vi "知乎日报.vi"() -> ()   [LabVIEW 2012]
panel:
  in  "关于作者":bool
  in  "刷新":bool
  out "stories":T1(array[cluster])
  out "top_stories":cluster{"字符串 2":string, "二维图片":picture}[](array[cluster])
  out "title with pic":cluster{"字符串 2":string, "二维图片":picture}[](array[cluster])
  in  "WebBrowser":refnum<k7>(container) caption="网页浏览器"
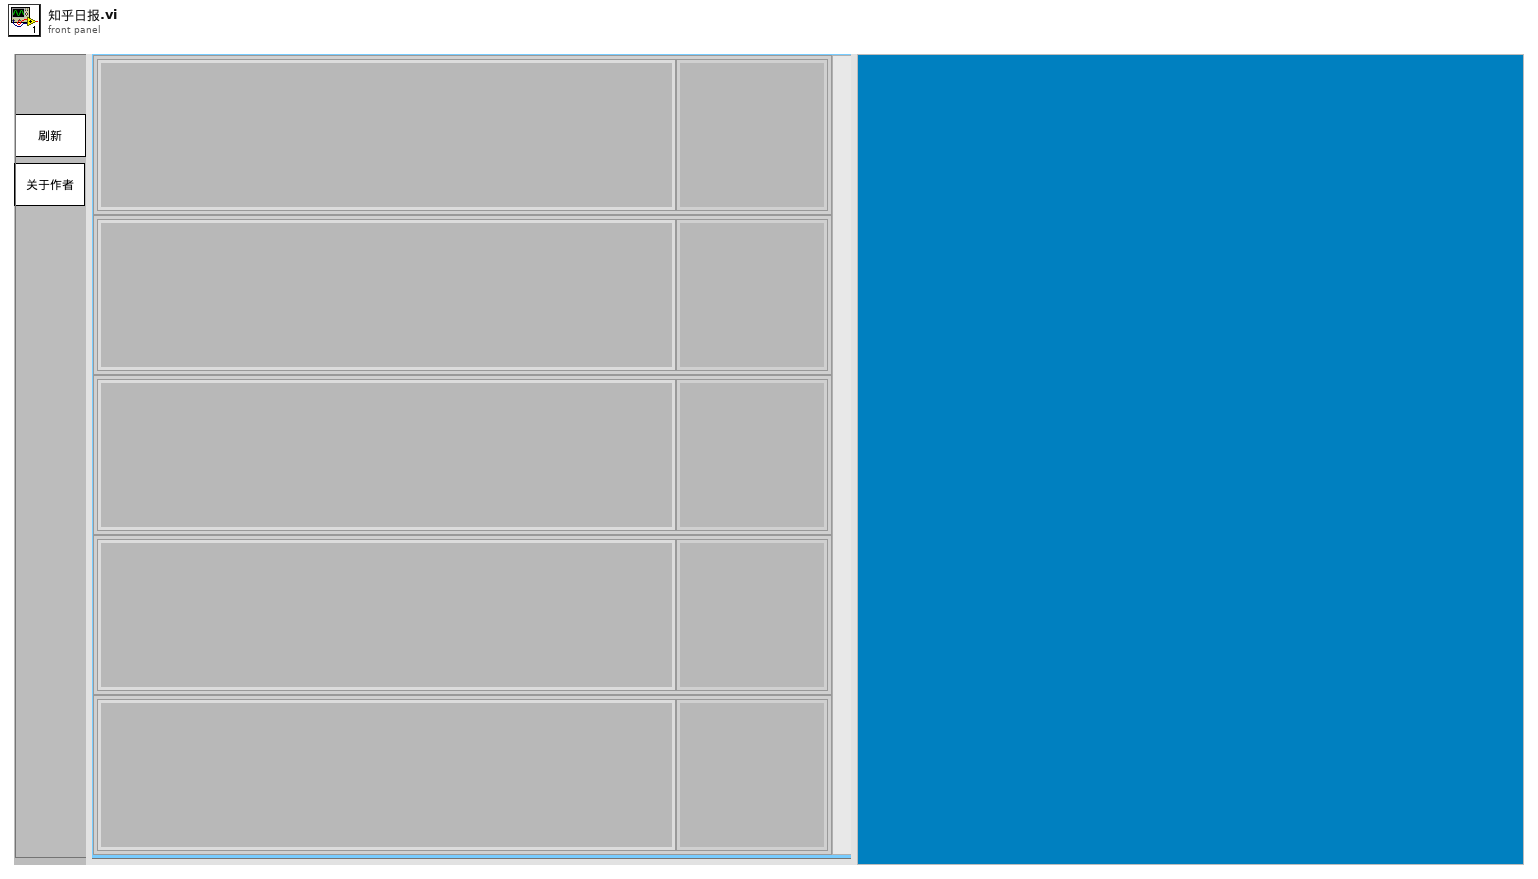
[diagram p1: front panel]
types:
  T1 = cluster{"images":string, "type":i32, "id":i64, "ga_prefix":string, "title":string}[]
  T2 = cluster{"images":string, "type":i32, "id":i64, "ga_prefix":string, "title":string}
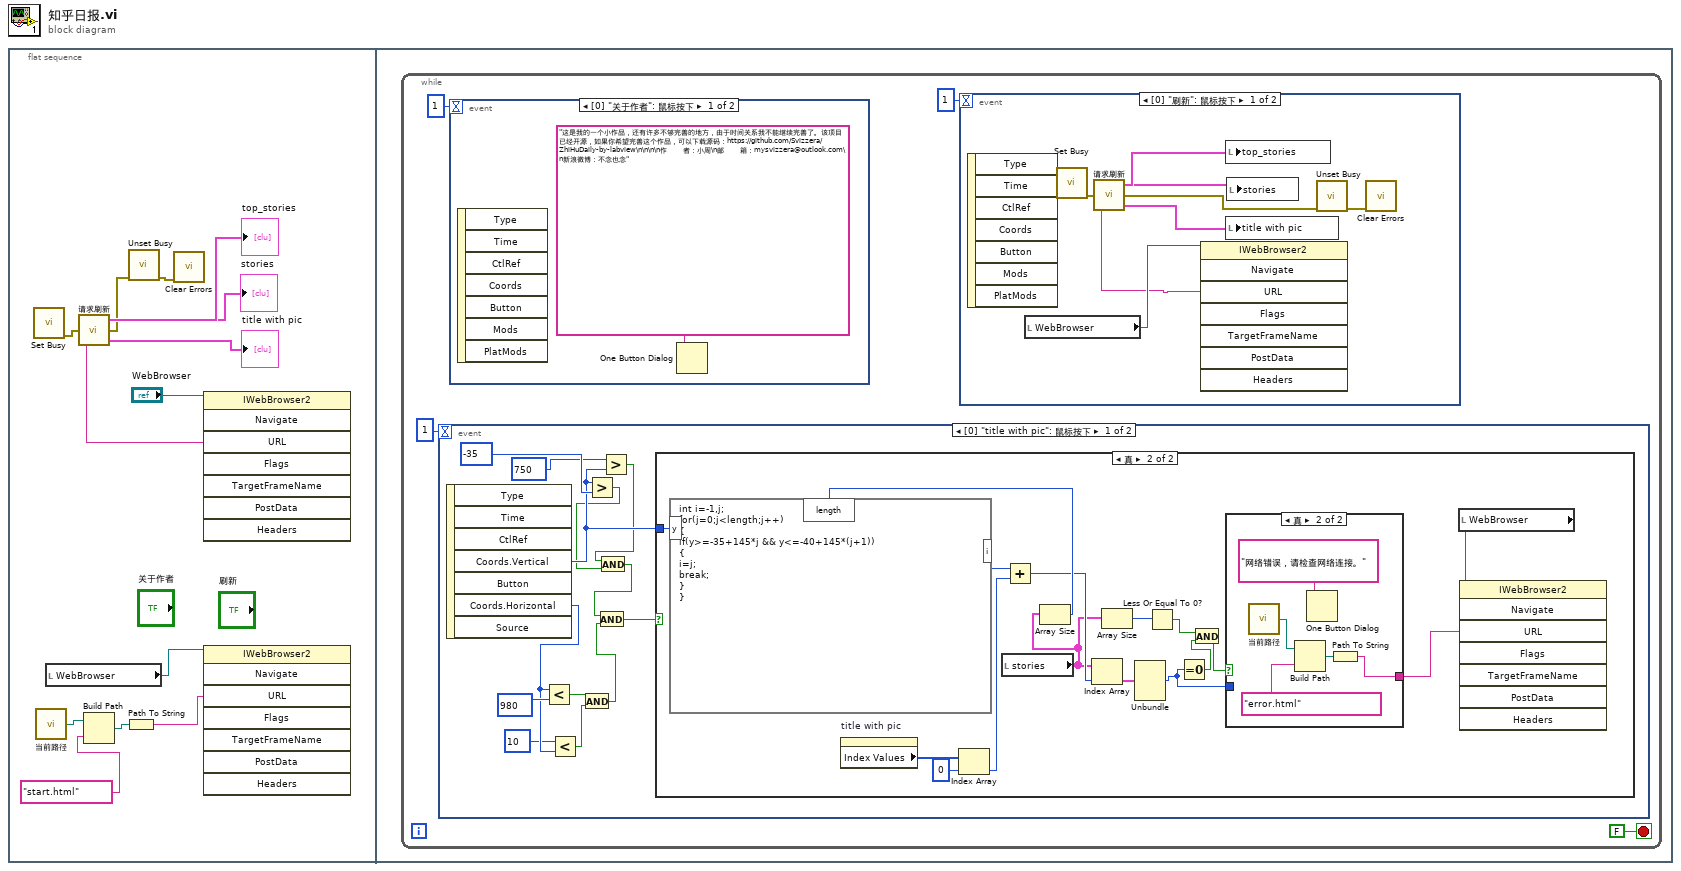
[diagram p0: block diagram]
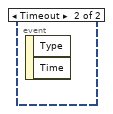
[diagram p2: hidden frame]
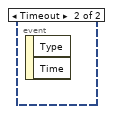
[diagram p3: hidden frame]
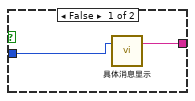
[diagram p5: hidden frame]
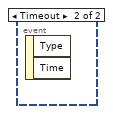
[diagram p6: hidden frame]
diagram:
  n1 = flat-sequence {
    frame #0 {
      n2 = call <vilib>:"Set Busy.vi"() -> ("error out"=w9:errorcluster)  [unwired: 10 in, 1 out]
      n3 = call "当前路径.vi"() -> ("路径"=w4:path)
      n4 = local read "WebBrowser"() -> (w5:refnum<k7>)
      n5 = call "请求刷新.vi"("Error Out"=w9) -> ("title with pic"=→"title with pic":cluster{"字符串 2":string, "二维图片":picture}[], "error out"=w7:errorcluster, "stories"=→"stories":T1, "URL"=w6:string, "top_stories"=→"top_stories":cluster{"字符串 2":string, "二维图片":picture}[])
      n6 = Build Path(base path=w4, name or relative path="start.html") -> (appended path=w2:path)
      n7 = Path To String(path=w2) -> (string=w1:string)
      n8 = call <vilib>:"Unset Busy.vi"("error in (no error)"=w7) -> ("error out"=w8:errorcluster)  [unwired: 10 in]
      n9 = call <vilib>:"Clear Errors.vi"("error in (no error)"=w8) -> ()  [unwired: 6 in, 1 out]
      n10 = invoke class="IWebBrowser2" method="Navigate"(reference="WebBrowser", "URL"=w6) -> ()  [unwired: 6 in, 8 out]
      n11 = invoke class="IWebBrowser2" method="Navigate"(reference=w5, "URL"=w1) -> ()  [unwired: 6 in, 8 out]
    }
    frame #1 {
      n12 = while {
        stop <- FALSE stop-if-true
        n13 = event shown="[0] \"title with pic\": 鼠标按下" {
          selector: _ -> [_ _]
          dyn-events: _ -> [_ _]
          timeout: 1 -> [_ _]
          event "title with pic": Mouse Down {
            n14 = event-data() -> ("Coords.Vertical"=w36:i32, "Coords.Horizontal"=w31:i32)  [unwired: 1 in, 5 out]
            n15 = Less?(x=w31, y=980) -> (x < y?=w29:bool)
            n16 = Less?(x=10, y=w31) -> (x < y?=w28:bool)
            n17 = And(x=w29, y=w28) -> (x .and. y?=w27:bool)
            n18 = Greater?(x=w36, y=-35) -> (0:w33:bool)
            n19 = Greater?(x=750, y=w36) -> (0:w34:bool)
            n20 = And(x=w34, y=w33) -> (x .and. y?=w32:bool)
            n21 = And(x=w32, y=w27) -> (x .and. y?=w37:bool)
            n22 = case shown="真" w37 {
              tunnel: w36 -> [_ w48]
              frame False {
              }
              frame True {
                n23 = property on="title with pic" class="Arr (严格)"() -> ("Index Values"=w51:u32[])  [unwired: 2 in, 2 out]
                n24 = Index Array(array=w51, index=0) -> (element=w49:u32)
                n25 = local read "stories"() -> (w45:T1)
                n26 = Array Size(array=w45) -> (size(s)=w53:i32)
                n27 = formula code="int i=-1,j;\nfor(j=0;j<length;j++)\n{\nif(y>=-35+145*j && y<=-40+145*(j+1))\n{\ni=j;\nbreak;\n}\n}"("y"=w48, "length"=w53) -> ("i"=w52:i32)
                n28 = Add(x=w52, y=w49) -> (x+y=w47:u32)
                n29 = Index Array(array=w45, index=w47) -> (element=w46:T2)
                n30 = Array Size(array=w45) -> (size(s)=w44:i32)
                n31 = Unbundle(w46) -> ("id"=w54:i64)  [unwired: 4 out]
                n32 = Less Or Equal To 0?(x=w44) -> (x <= 0?=w42:bool)
                n33 = Equal To 0?(x=w54) -> (x = 0?=w41:bool)
                n34 = And(x=w42, y=w41) -> (x .and. y?=w43:bool)
                n35 = case shown="真" w43 {
                  tunnel: w54 -> [w57 _]
                  tunnel: [w56 w58] -> w40
                  frame False {
                    n36 = call "具体消息显示.vi"("ID"=w57) -> ("html_url"=w56:string)  [unwired: 2 in]
                  }
                  frame True {
                    n37 = call "当前路径.vi"() -> ("路径"=w60:path)
                    n38 = Build Path(base path=w60, name or relative path="error.html") -> (appended path=w62:path)
                    n39 = One Button Dialog(message="网络错误，请检查网络连接。") -> ()  [unwired: 1 in, 1 out]
                    n40 = Path To String(path=w62) -> (string=w58:string)
                  }
                }
                n41 = local read "WebBrowser"() -> (w55:refnum<k7>)
                n42 = invoke class="IWebBrowser2" method="Navigate"(reference=w55, "URL"=w40) -> ()  [unwired: 6 in, 8 out]
              }
            }
          }
          event Timeout {
            n43 = event-data() -> ()  [unwired: 1 in, 2 out]
          }
        }
        n44 = event shown="[0] \"关于作者\": 鼠标按下" {
          selector: _ -> [_ _]
          dyn-events: _ -> [_ _]
          timeout: 1 -> [_ _]
          event "关于作者": Mouse Down {
            n45 = event-data() -> ()  [unwired: 1 in, 7 out]
            n46 = One Button Dialog(message="这是我的一个小作品，还有许多不够完善的地方，由于时间关系我不能继续完善了。该项目已经开源，如果你希望完善这个作品，可以下载源码：https://github.com/Svizzera/ZhiHuDaily-by-labview\n\n\n\n作        者：小周\n邮        箱：mysvizzera@outlook.com\n新浪微博：不念也念") -> ()  [unwired: 1 in, 1 out]
          }
          event Timeout {
            n47 = event-data() -> ()  [unwired: 1 in, 2 out]
          }
        }
        n48 = event shown="[0] \"刷新\": 鼠标按下" {
          selector: _ -> [_ _]
          dyn-events: _ -> [_ _]
          timeout: 1 -> [_ _]
          event "刷新": Mouse Down {
            n49 = event-data() -> ()  [unwired: 1 in, 7 out]
            n50 = local read "WebBrowser"() -> (w25:refnum<k7>)
            n51 = call <vilib>:"Set Busy.vi"() -> ("error out"=w20:errorcluster)  [unwired: 10 in, 1 out]
            n52 = call "请求刷新.vi"("Error Out"=w20) -> ("title with pic"=w22:cluster{"字符串 2":string, "二维图片":picture}[], "error out"=w19:errorcluster, "stories"=w23:T1, "URL"=w18:string, "top_stories"=w24:cluster{"字符串 2":string, "二维图片":picture}[])
            n53 = invoke class="IWebBrowser2" method="Navigate"(reference=w25, "URL"=w18) -> ()  [unwired: 6 in, 8 out]
            n54 = local write "top_stories"(w24) -> ()
            n55 = local write "title with pic"(w22) -> ()
            n56 = local write "stories"(w23) -> ()
            n57 = call <vilib>:"Unset Busy.vi"("error in (no error)"=w19) -> ("error out"=w21:errorcluster)  [unwired: 10 in]
            n58 = call <vilib>:"Clear Errors.vi"("error in (no error)"=w21) -> ()  [unwired: 6 in, 1 out]
          }
          event Timeout {
            n59 = event-data() -> ()  [unwired: 1 in, 2 out]
          }
        }
      }
    }
  }
